vi "Generate Unique Header.vi"(8 "error in (no error)":errorcluster, 11 "PAS Cell Data in":refnum<class "PAS Cell Data.lvclass">) -> (0 "error out":errorcluster, 2 "Header":string[](array[string]), 3 "PAS Cell Data out":refnum<class "PAS Cell Data.lvclass">)   [LabVIEW 2014, in "PAS Cell Data.lvclass"]
uses:
  PAS Cell Data.lvclass
  Data/Data.lvclass/Data.ctl
  Data/Read Data ID.vi
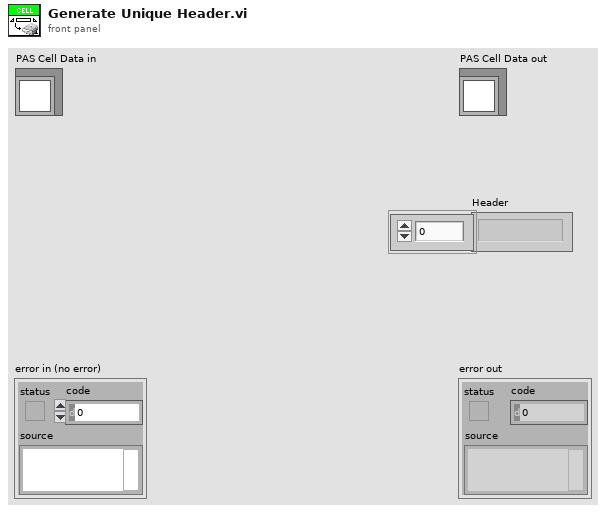
[diagram p1: front panel]
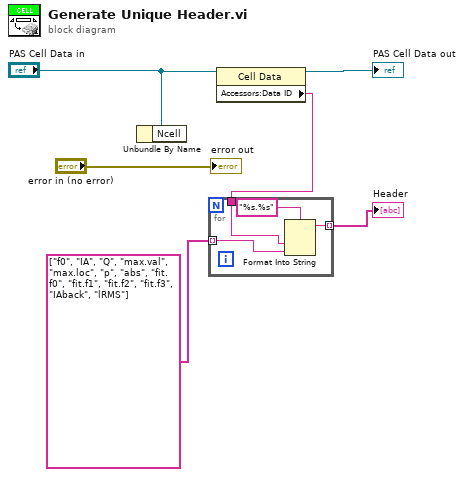
[diagram p0: block diagram]
diagram:
  n1 = Unbundle By Name("PAS Cell Data in") -> ()  [unwired: 1 out]
  n2 = property class="Cell Data"(reference="PAS Cell Data in") -> (reference out=→"PAS Cell Data out":refnum<class "PAS Cell Data.lvclass">, "Accessors:Data ID"=w1:string)  [unwired: 1 in, 1 out]
  n3 = for {
    tunnel: string[] ["f0", "IA", "Q", "max.val", "max.loc", "p", "abs", "fit.f0", "fit.f1", "fit.f2", "fit.f3", "IAback", "lRMS"] -> [w10] mode=indexing
    tunnel: [w8] -> w4 mode=indexing
    tunnel: w1 -> [w7]
    n4 = Format Into String(format string="%s.%s", w7, w10) -> (resulting string=w8:string)  [unwired: 2 in, 1 out]
  }
  "Header" <- w4
  "error out" <- "error in (no error)"
